vi "Work1.vi"(8 "Boolean":bool, 10 "B":dbl, 11 "A":dbl) -> (2 "Resaly":dbl)   [LabVIEW 2020]
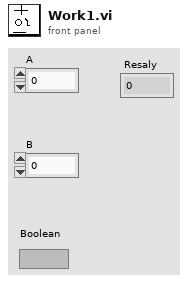
[diagram p1: front panel]
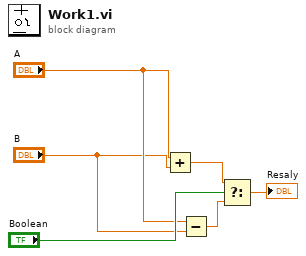
[diagram p0: block diagram]
diagram:
  n1 = Add(x="A", y="B") -> (x+y=w5:dbl)
  n2 = Subtract(x="A", y="B") -> (x-y=w4:dbl)
  n3 = Select(t=w5, s="Boolean", f=w4) -> (s? t:f=→"Resaly":dbl)
